vi "Display Uploaded Mission Waypoints.vi"(7 "Aircraft ID":u8, 8 "Error In":errorcluster, 11 "Waypoints":T1[](array[typedef])) -> (0 "Error Out":errorcluster)   [LabVIEW 2014]
uses:
  C:/Robotic Systems/Products/Surveyor/Software/Ground Station/Data/Mapping DLL/GMap.NET.WindowsForms.dll
  Data/Mapping DLL/GMap.NET.WindowsForms.dll
  MAVLink/Controls/Mission Planning Controls/MAVLINK Mission Item.ctl
  MAVLink/Controls/MAVLINK Mav Frame.ctl
  Missions/Controls/Waypoint Type.ctl
  MAVLink/Waypoint Controller/FGV/Methods/Get Waypoint type.vi
  MAVLink/Waypoint Controller/FGV/Methods/Set Waypoint type.vi
panel:
  in  "Ok":bool
  in  "GMapControl":refnum<k24>(container)
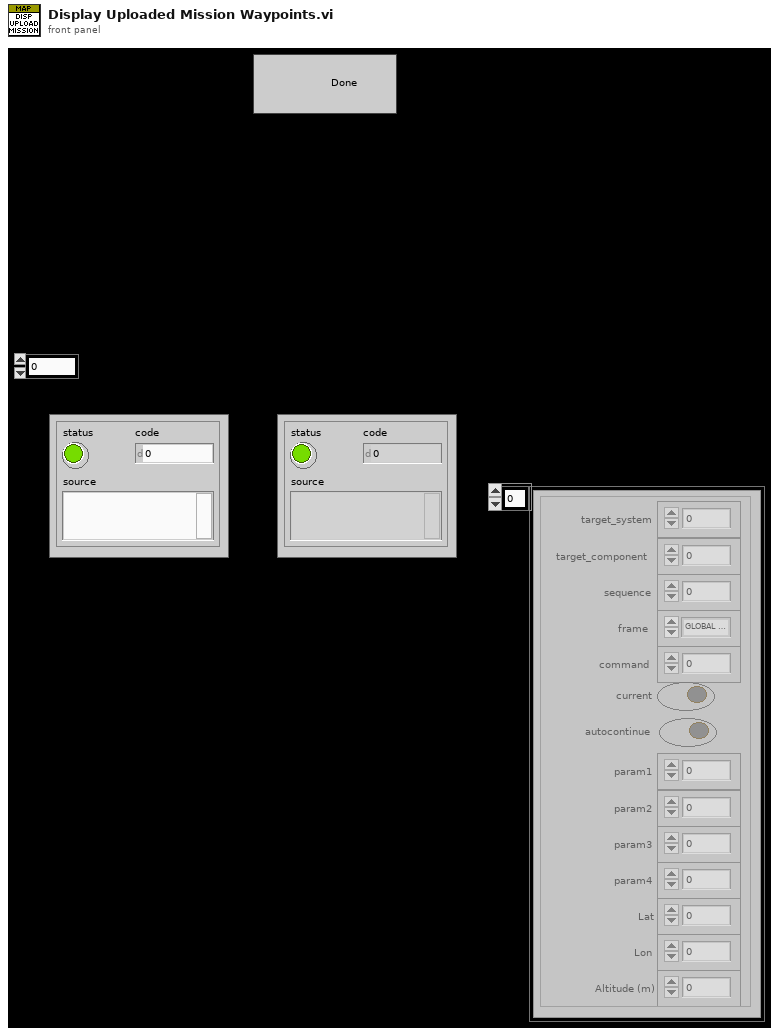
[diagram p1: front panel]
types:
  T1 = typedef "MAVLINK Mission Item.ctl" = cluster{"target_system":u8, "target_component":u8, "sequence":u16, "frame":T2, "command":u16, "current":bool, "autocontinue":bool, "param1":sgl, "param2":sgl, "param3":sgl, "param4":sgl, "Lat":sgl, "Lon":sgl, "Altitude (m)":sgl}
  T2 = typedef "MAVLINK Mav Frame.ctl" = enum8{"GLOBAL", "LOCAL NED", "MISSION", "GLOBAL RELATIVE ALT", "LOCAL ENU", "GLOBAL INT", "GLOBAL RELATIVE ALT INT", "LOCAL OFFSET NED", "BODY NED", "BODY OFFSET NED", "GLOBAL TERRAIN ALT", "GLOBAL TERRAIN ALT INT"}
  T3 = typedef "Waypoint Type.ctl" = enum16{"Pass-Through", "Inspect", "Circumnavigate"}
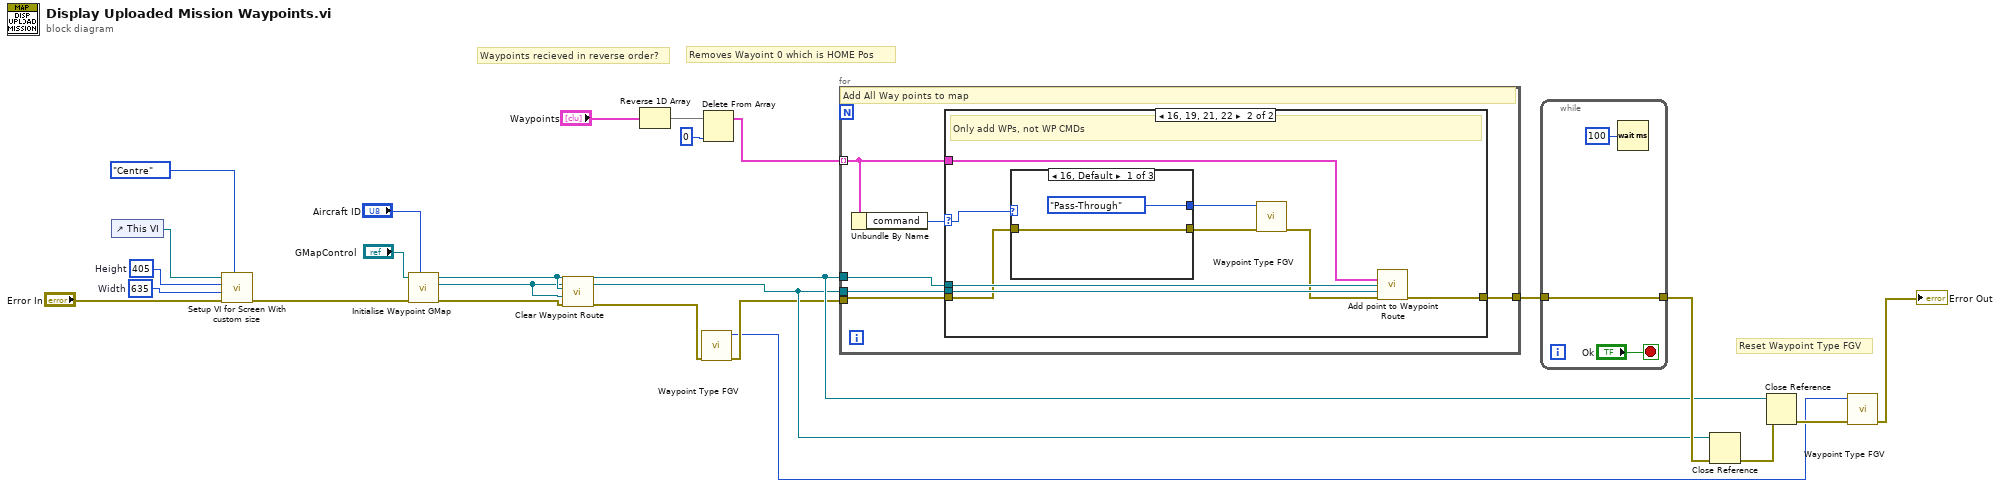
[diagram p0: block diagram]
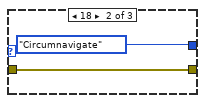
[diagram p3: hidden frame]
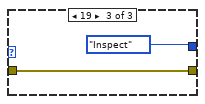
[diagram p4: hidden frame]
diagram:
  w7 = i16 635  # Width
  w8 = i16 405  # Height
  # "Reset Waypoint Type FGV"
  # "Waypoints recieved in reverse order?"
  # "Removes Wayoint 0 which is HOME Pos"
  n1 = control-ref of="This VI"() -> (w10:refnum<vi>)
  n2 = call "Setup VI for Screen With custom size.vi"("Position"=enum16{"Top Left", "Centre"}."Centre", "Error In"="Error In", "Width"=w7, "Height"=w8, "This VI"=w10) -> ("Error Out"=w6:errorcluster)  [unwired: 5 in, 1 out]
  n3 = call "Initialise Waypoint GMap.vi"("Aircraft ID"="Aircraft ID", "error in (no error)"=w6, "Main Map"="GMapControl") -> ("Error Out"=w18:errorcluster, "Main Map Control Ref"=w16:refnum<k24>, "Main map DLL Ref"=w17:refnum<k24>)  [unwired: 6 in]
  n4 = call "Clear Waypoint Route.vi"("Error In"=w18, "Main Map Reference"=w16, "Main Map DLL Ref"=w17) -> ("error out"=w5:errorcluster)  [unwired: 8 in]
  n5 = Reverse 1D Array(array="Waypoints") -> (reversed array=w14:T1[])
  n6 = call-poly "Waypoint Type FGV.vi"("Error In"=w5) -> ("Error Out"=w4:errorcluster, "Waypoint Type Out"=w1:T3)  [unwired: 9 in]
  n7 = Delete From Array(array=w14, index=0) -> (array with subset deleted=w12:T1[])  [unwired: 1 in, 1 out]
  n8 = for {
    tunnel: w12 -> [w25] mode=indexing
    tunnel: w4 -> [w27]
    tunnel: w17 -> [w29]
    tunnel: w16 -> [w28]
    tunnel: [w26] -> w21
    # "Add All Way points to map"
    n9 = Unbundle By Name(w25) -> ("command"=w24:u16)
    n10 = case shown="16, 19, 21, 22" w24 {
      selector: w24 -> [_ w35]
      tunnel: w29 -> [_ w39]
      tunnel: w28 -> [_ w38]
      tunnel: w27 -> [w30 w34]
      tunnel: [w30 w37] -> w26
      tunnel: w25 -> [_ w36]
      frame 115, 201, Default {
        # "Dont add ROI WPs"
      }
      frame 16, 19, 21, 22 {
        # "Only add WPs, not WP CMDs"
        n11 = case shown="16, Default" w35 {
          tunnel: w34 -> [w41 w42 w44]
          tunnel: [w41 w42 w44] -> w32
          tunnel: [Waypoint_Type."Pass-Through" ("Waypoint Type In") Waypoint_Type."Circumnavigate" ("Waypoint Type In") Waypoint_Type."Inspect" ("Waypoint Type In")] -> w31
          frame 16, Default {
          }
          frame 18 {
          }
          frame 19 {
          }
        }
        n12 = call-poly "Waypoint Type FGV.vi"("Error In"=w32, "Waypoint Type In"=w31) -> ("Error Out"=w33:errorcluster)  [unwired: 9 in]
        n13 = call "Add point to Waypoint Route.vi"("MISSION_ITEM"=w36, "Main Map DLL Ref"=w39, "Main Map Control Reference"=w38, "Error In"=w33) -> ("Error Out"=w37:errorcluster)  [unwired: 11 in]
      }
    }
  }
  n14 = while {
    tunnel: w21 -> [w46]
    tunnel: [w46] -> w19
    stop <- "Ok" stop-if-true
    n15 = Wait (ms)(milliseconds to wait=u32 100) -> ()  [unwired: 1 out]
  }
  n16 = Close Reference(reference=w16, error in (no error)=w19) -> (error out=w20:errorcluster)
  n17 = Close Reference(reference=w17, error in (no error)=w20) -> (error out=w3:errorcluster)
  n18 = call-poly "Waypoint Type FGV.vi"("Error In"=w3, "Waypoint Type In"=w1) -> ("Error Out"=→"Error Out":errorcluster)  [unwired: 9 in]
